vi "flipY.vi"(11 "Array in":cluster{"a":dbl, dbl}[](array[cluster])) -> (3 "Array out":cluster{"a":dbl, dbl}[](array[cluster]))   [LabVIEW 2022 SP3]
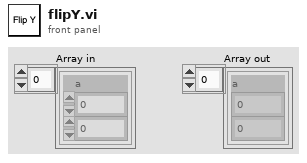
[diagram p1: front panel]
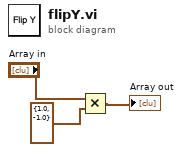
[diagram p0: block diagram]
diagram:
  n1 = Multiply(x="Array in", y=cluster{"a":dbl, dbl} {"a"=1.0, -1.0}) -> (x*y=→"Array out":cluster{"a":dbl, dbl}[])
